vi "test read variatn.vi"() -> ()   [LabVIEW 2020, in "ThorlabsWavefrontDS.lvclass"]
uses:
  ThorlabsWavefrontDS.lvclass
panel:
  out "values":dbl
  out "data":variant
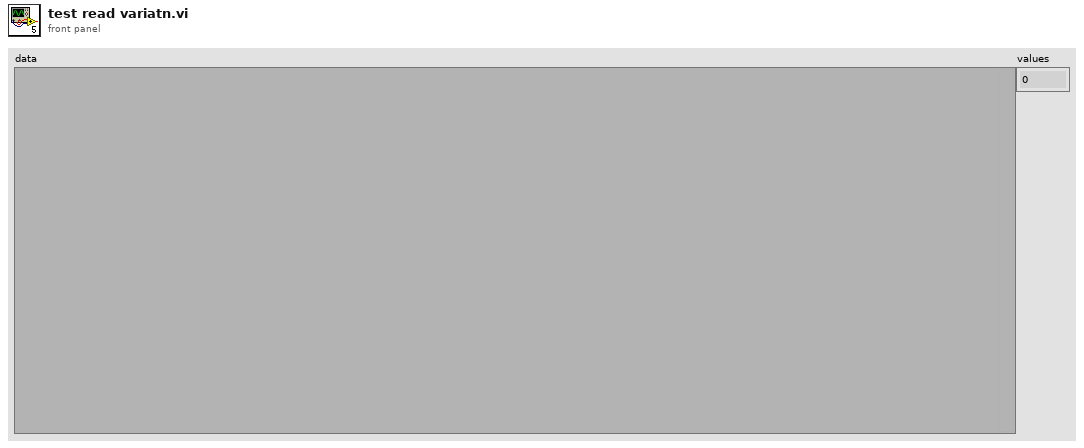
[diagram p1: front panel]
types:
  T1 = enum16{"Read", "Write", "ReadWrite", "BufferedRead", "BufferedReadWrite"}
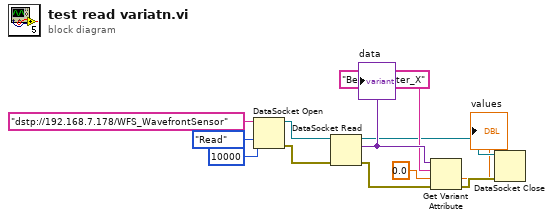
[diagram p0: block diagram]
diagram:
  n1 = DataSocket Open(9:10000 ("ms timeout (10000)"), 10:T1."Read" ("mode"), 11:"dstp://192.168.7.178/WFS_WavefrontSensor" ("URL")) -> (0:w4:errorcluster, 3:w7:refnum<k13>)  [unwired: 1 in]
  n2 = DataSocket Read(8:w4, 11:w7) -> (0:w11:errorcluster, 2:w12:variant, 3:w6:refnum<k13>)  [unwired: 3 in, 4 out]
  "data" <- w12
  n3 = Get Variant Attribute(Variant=w12, name="Beam_Center_X", default value (empty Variant)=0.0, error in=w11) -> (value=→"values":dbl, error out=w5:errorcluster)  [unwired: 2 out]
  n4 = DataSocket Close(8:w5, 11:w6) -> ()  [unwired: 1 in, 2 out]
